vi "Measurement.SetConfiguration.vi"(8 "error in (no error)":errorcluster, 10 "Configuration":variant, 11 "Measurement.IVCurve in":refnum<class "Measurement.IVCurve.lvclass">) -> (0 "error out":errorcluster, 3 "Measurement.IVCurve out":refnum<class "Measurement.IVCurve.lvclass">)   [LabVIEW 2019, in "Measurement.IVCurve.lvclass"]
uses:
  Measurement.IVCurve.lvclass
  Typedefs/Configuration--Cluster.ctl
  Measurement/Typedefs/Measurement.Type--Enum.ctl
  Typedefs/Configuration.Hardware--Cluster.ctl
  Measurement/Typedefs/Configuration.SMU--Cluster.ctl
  SMU/Typedefs/Configuration--Cluster.ctl
  Typedefs/Configuration.Measurement--Cluster.ctl
  Measurement/Measurement.lvclass
  SMU/SMU.lvclass
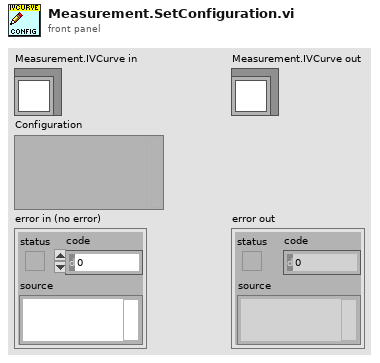
[diagram p1: front panel]
types:
  T1 = typedef "Measurement.IVCurve.lvclass/Configuration--Cluster.ctl" = cluster{"Measurement.Type":T2, "Hardware":T3, "Measurement":T6}
  T2 = typedef "Measurement.lvclass/Measurement.Type--Enum.ctl" = enum16{"Free", "I/V Curve", "Wavelength sweeping", "Photocurrent mapping"}
  T3 = typedef "Measurement.IVCurve.lvclass/Configuration.Hardware--Cluster.ctl" = cluster{"SMU":T4}
  T4 = typedef "Measurement.lvclass/Configuration.SMU--Cluster.ctl" = cluster{"Enable":bool, "SMU Model":string, "Configuration":T5}
  T5 = typedef "SMU.lvclass/Configuration--Cluster.ctl" = cluster{"VISA Resource":string, "Channel":string}
  T6 = typedef "Measurement.IVCurve.lvclass/Configuration.Measurement--Cluster.ctl" = cluster{"SMU Voltage Start, V":dbl, "SMU Voltage Stop, V":dbl, "SMU Voltage Step, V":dbl, "Delay time, ms":u16, "Accumulation":u16}
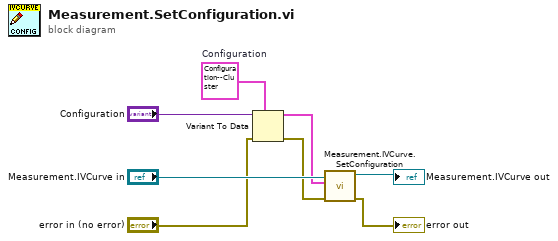
[diagram p0: block diagram]
diagram:
  w7 = T1 {"Measurement.Type"=enum."Free", "Hardware"={"SMU"={"Enable"=FALSE, "SMU Model"="", "Configuration"={"VISA Resource"="", "Channel"=""}}}, "Measurement"={"SMU Voltage Start, V"=0.0, "SMU Voltage Stop, V"=0.0, "SMU Voltage Step, V"=0.0, "Delay time, ms"=0, "Accumulation"=0}}  # Configuration
  n1 = Variant To Data(error in="error in (no error)", type=w7, Variant="Configuration") -> (data=w4:T1, error out=w3:errorcluster)
  n2 = call "Measurement.IVCurve.SetConfiguration.vi"("error in (no error)"=w3, "Configuration"=w4, "Measurement.IVCurve"="Measurement.IVCurve in") -> ("error out"=→"error out":errorcluster, "Measurement.IVCurve out"=→"Measurement.IVCurve out":refnum<class "Measurement.IVCurve.lvclass">)  [unwired: 7 in]
